vi "mainog.vi"() -> ()   [LabVIEW 2014]
uses:
  <vilib>/Instr/_visa.llb/VISA Configure Serial Port (Instr).vi
panel:
  in  "Write Pressure Values":bool
  in  "Keep Data?":bool
  out "12bit DAC signal sent":string
  in  "filepath:":path
  out "Pressure Plot":i32[](graph)
  in  "Desired Pressures":dbl[](array[numeric])
  out "mbar":string[](array[string])
  out "status":bool
  out "error out":errorcluster
  in  "error in":errorcluster
  in  "stop":bool
  # "Arduino LabVIEW - Serial Read and Write"
  # "Measured Pressures"
  # "Desired pressures must be expressed in volts (0-5)"
  # "Channel 1"
  # "Channel 2"
  # "Channel 1"
  # "Channel 3"
  # "Channel 2"
  # "Channel 4"
  # "Channel 3"
  # "Channel 4"
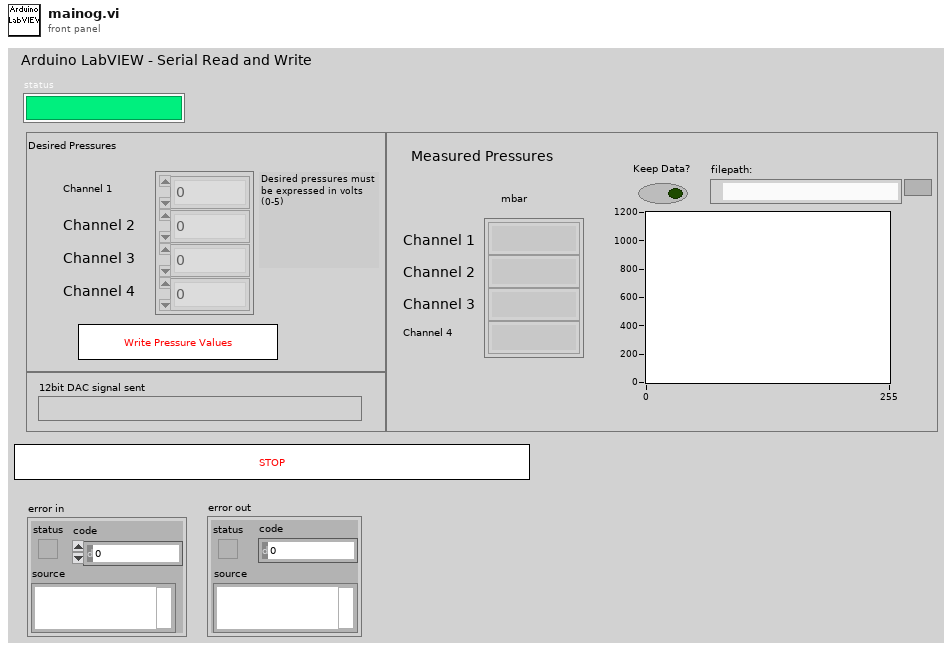
[diagram p1: front panel]
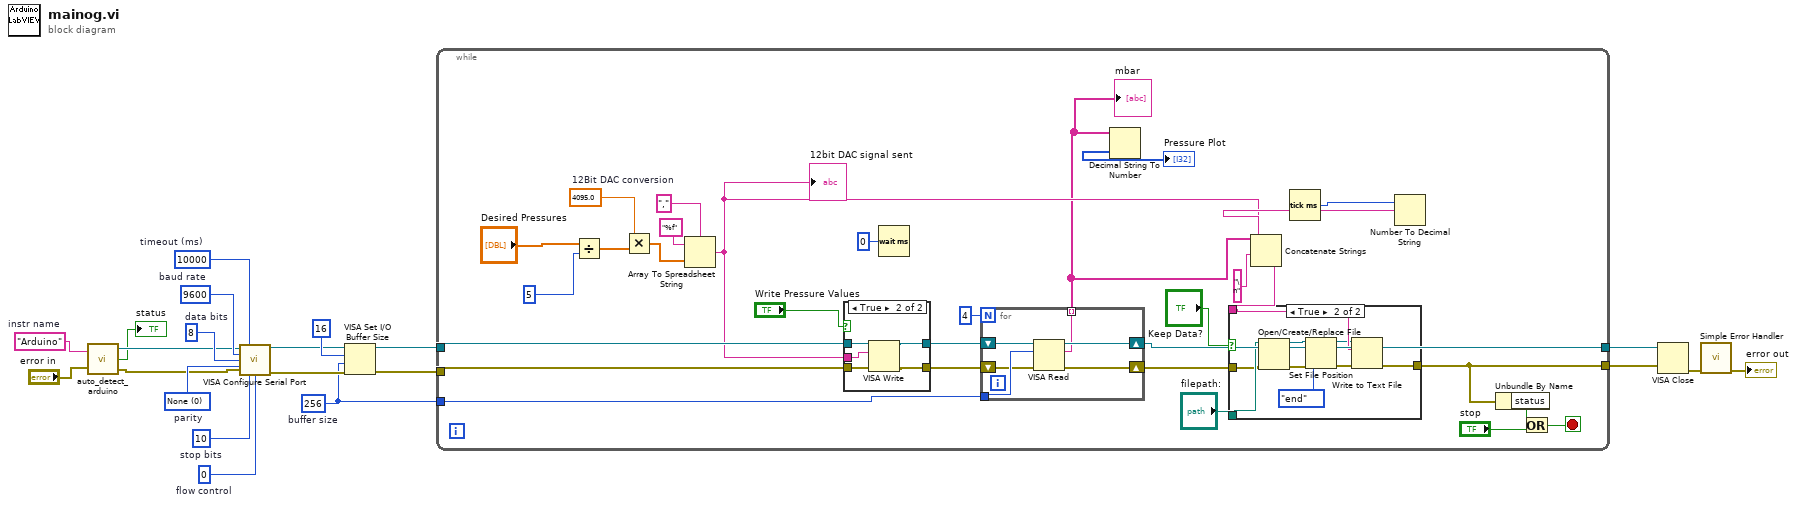
[diagram p0: block diagram]
diagram:
  w12 = "Arduino"  # instr name
  w6 = u32 256  # buffer size
  w19 = u16 0  # flow control
  w18 = u16 10  # stop bits
  w17 = u16 0 items=["None", "Odd", "Even", "Mark", "Space"]  # parity
  w16 = u16 8  # data bits
  w15 = u32 9600  # baud rate
  w20 = u32 10000  # timeout (ms)
  n1 = call "auto_detect_arduino.vi"("instr name"=w12, "error in"="error in") -> ("VISA resource name"=w14:refnum<visa-resource-name>, "status"=→"status":bool, "error out"=w13:errorcluster)
  n2 = call-poly "VISA Configure Serial Port"("VISA resource name"=w14, "timeout (10sec)"=w20, "baud rate (9600)"=w15, "data bits (8)"=w16, "parity (0:none)"=w17, "error in (no error)"=w13, "stop bits (10: 1 bit)"=w18, "flow control (0:none)"=w19) -> ("VISA resource name out"=w10:refnum<visa-resource-name>, "error out"=w9:errorcluster)  [unwired: 6 in]
  n3 = VISA Set I/O Buffer Size(VISA resource name=w10, mask (16)=u16 16 ("I/O Receive\nBuffer mask"), size (4096)=w6, error in (no error)=w9) -> (VISA resource name out=w8:refnum<visa-resource-name>, error out=w7:errorcluster)
  n4 = while {
    tunnel: w8 -> [w47]
    tunnel: w7 -> [w46]
    tunnel: [w48] -> w21
    tunnel: w6 -> [w49]
    tunnel: [w32] -> w1
    stop <- w50 stop-if-true
    w35 = 4095.0  # 12Bit DAC conversion
    n5 = Divide(x="Desired Pressures", y=5) -> (x/y=w37:dbl[])
    n6 = Multiply(x=w35, y=w37) -> (x*y=w36:dbl[])
    n7 = Array To Spreadsheet String(delimiter (Tab)=",", array=w36, 3:"%f" ("format string")) -> (spreadsheet string=w24:string)
    "12bit DAC signal sent" <- w24
    n8 = case shown="True" "Write Pressure Values" {
      tunnel: w47 -> [w69 w74]
      tunnel: w46 -> [w68 w73]
      tunnel: [w69 w72] -> w45
      tunnel: [w68 w71] -> w44
      tunnel: w24 -> [_ w70]
      frame False {
      }
      frame True {
        n9 = VISA Write(VISA resource name=w74, write buffer=w70, error in (no error)=w73) -> (VISA resource name out=w72:refnum<visa-resource-name>, error out=w71:errorcluster)  [unwired: 1 out]
      }
    }
    n10 = Wait (ms)(milliseconds to wait=u32 0) -> ()  [unwired: 1 out]
    n11 = for {
      N: 4 -> [_]
      tunnel: w49 -> [w66]
      tunnel: [w62] -> w22 mode=indexing
      shift-right: [w65] -> w48
      shift-left: w45 -> [w64]
      shift-right: [w67] -> w33
      shift-left: w44 -> [w63]
      n12 = VISA Read(VISA resource name=w64, byte count=w66, error in (no error)=w63) -> (VISA resource name out=w65:refnum<visa-resource-name>, read buffer=w62:string, error out=w67:errorcluster)  [unwired: 1 out]
    }
    "mbar" <- w22
    n13 = Decimal String To Number(string=w22) -> (number=→"Pressure Plot":i32[])  [unwired: 2 in, 1 out]
    n14 = Tick Count (ms)() -> (millisecond timer value=w25:u32)
    n15 = Number To Decimal String(number=w25) -> (decimal integer string=w26:string)  [unwired: 1 in]
    n16 = Concatenate Strings(w22, w26, "\n" ("string"), w24) -> (w28:string)
    n17 = case shown="True" "Keep Data?" {
      tunnel: w28 -> [_ w61]
      tunnel: "filepath:" -> [_ w60]
      tunnel: w33 -> [w52 w59]
      tunnel: [w52 w54] -> w32
      frame False {
      }
      frame True {
        n18 = Open/Create/Replace File(file path (use dialog)=w60, error in=w59) -> (refnum out=w57:refnum<file>, error out=w58:errorcluster)  [unwired: 4 in, 1 out]
        n19 = Set File Position(refnum=w57, from (0:start)=enum16{"start", "end", "current"}."end", error in=w58) -> (refnum out=w56:refnum<file>, error out=w55:errorcluster)  [unwired: 1 in]
        n20 = Write to Text File(file (use dialog)=w56, text=w61, error in=w55) -> (error out=w54:errorcluster)  [unwired: 1 in, 2 out]
      }
    }
    n21 = Unbundle By Name(w32) -> ("status"=w31:bool)
    n22 = Or(x=w31, y="stop") -> (x .or. y?=w50:bool)
  }
  n23 = VISA Close(VISA resource name=w21, error in (no error)=w1) -> (error out=w4:errorcluster)
  n24 = call <vilib>:"Simple Error Handler.vi"("error in (no error)"=w4) -> ("error out"=→"error out":errorcluster)  [unwired: 4 in, 4 out]
